vi "sub_ubx-packet-final.vi"(11 "read_buffer":string) -> (1 "ubx arr":T1[](array[typedef]) {"class" format="%x"; "id" format="%x"; "len" format="%x"; "payload" format="%02x"; "chksum" format="%02x"; "next" format="%02x"}, 2 "latlong":cluster{dbl, dbl} {"?" format="%.8f"; "?" format="%.8f"}, 3 "val":bool)   [LabVIEW 2019]
uses:
  Ctrl/ubx-packet.ctl
  Ctrl/cmd_common.ctl
panel:
  out "RTK FIXED":bool
  in  "nav":enum32{"HPPOSLLH", "PVT", "DOP"}(tab)
  out "ubx-packet_hpposllh":T1 {"payload" format="%02x"; "chksum" format="%02x"; "next" format="%02x"}
  out "ubx-packet_pvt":T1 {"payload" format="%02x"; "chksum" format="%02x"; "next" format="%02x"}
  out "ubx-packet_dop":T1 {"payload" format="%02x"; "chksum" format="%02x"; "next" format="%02x"}
  out "str":string
  out "RTK FLOAT":bool
  out "flag":bool[](array[boolean])
  out "GNSSfix Type":u8
  out "ubz arr1":T1[](array[typedef]) {"payload" format="%02x"; "chksum" format="%02x"; "next" format="%02x"}
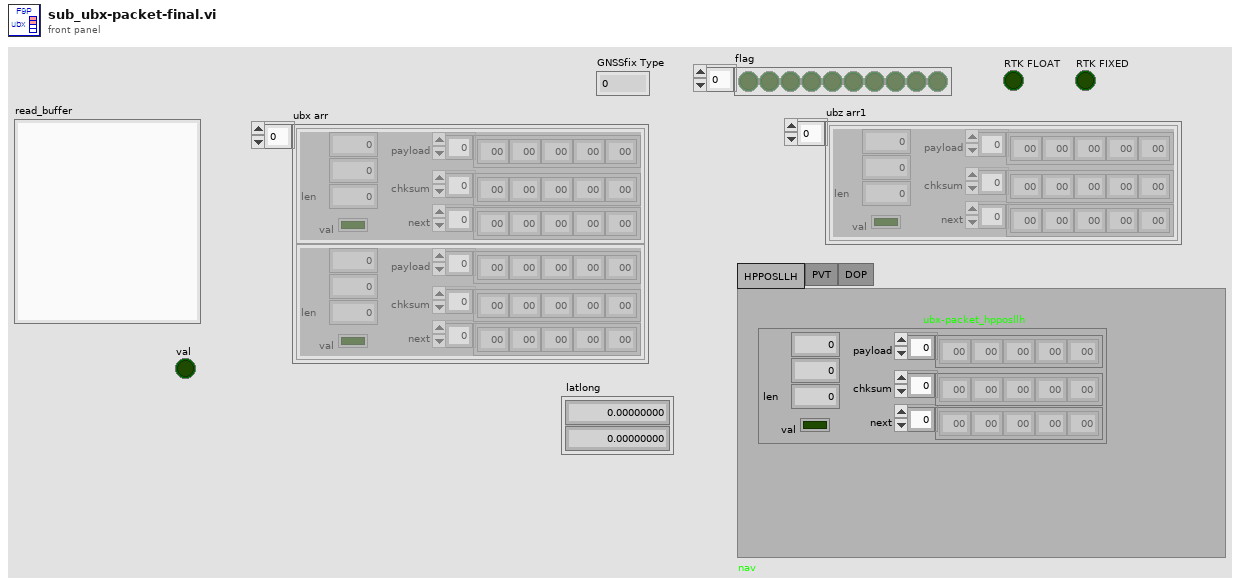
[diagram p1: front panel]
types:
  T1 = typedef "ubx-packet.ctl" = cluster{"class":u8, "id":u8, "len":u8, "payload":u8[], "chksum":u8[], "next ":u8[], "val":bool}
  T2 = typedef "cmd_common.ctl" = enum16{"read", "write"}
  T3 = typedef "ublox-ui_main.ctl" = cluster{"Longitude  ":dbl, "Latitude     ":dbl, "Fix Mode   ":string, "3D Acc.m":dbl, "2D Acc.m":dbl, "PDOP     ":dbl, "HDOP     ":dbl}
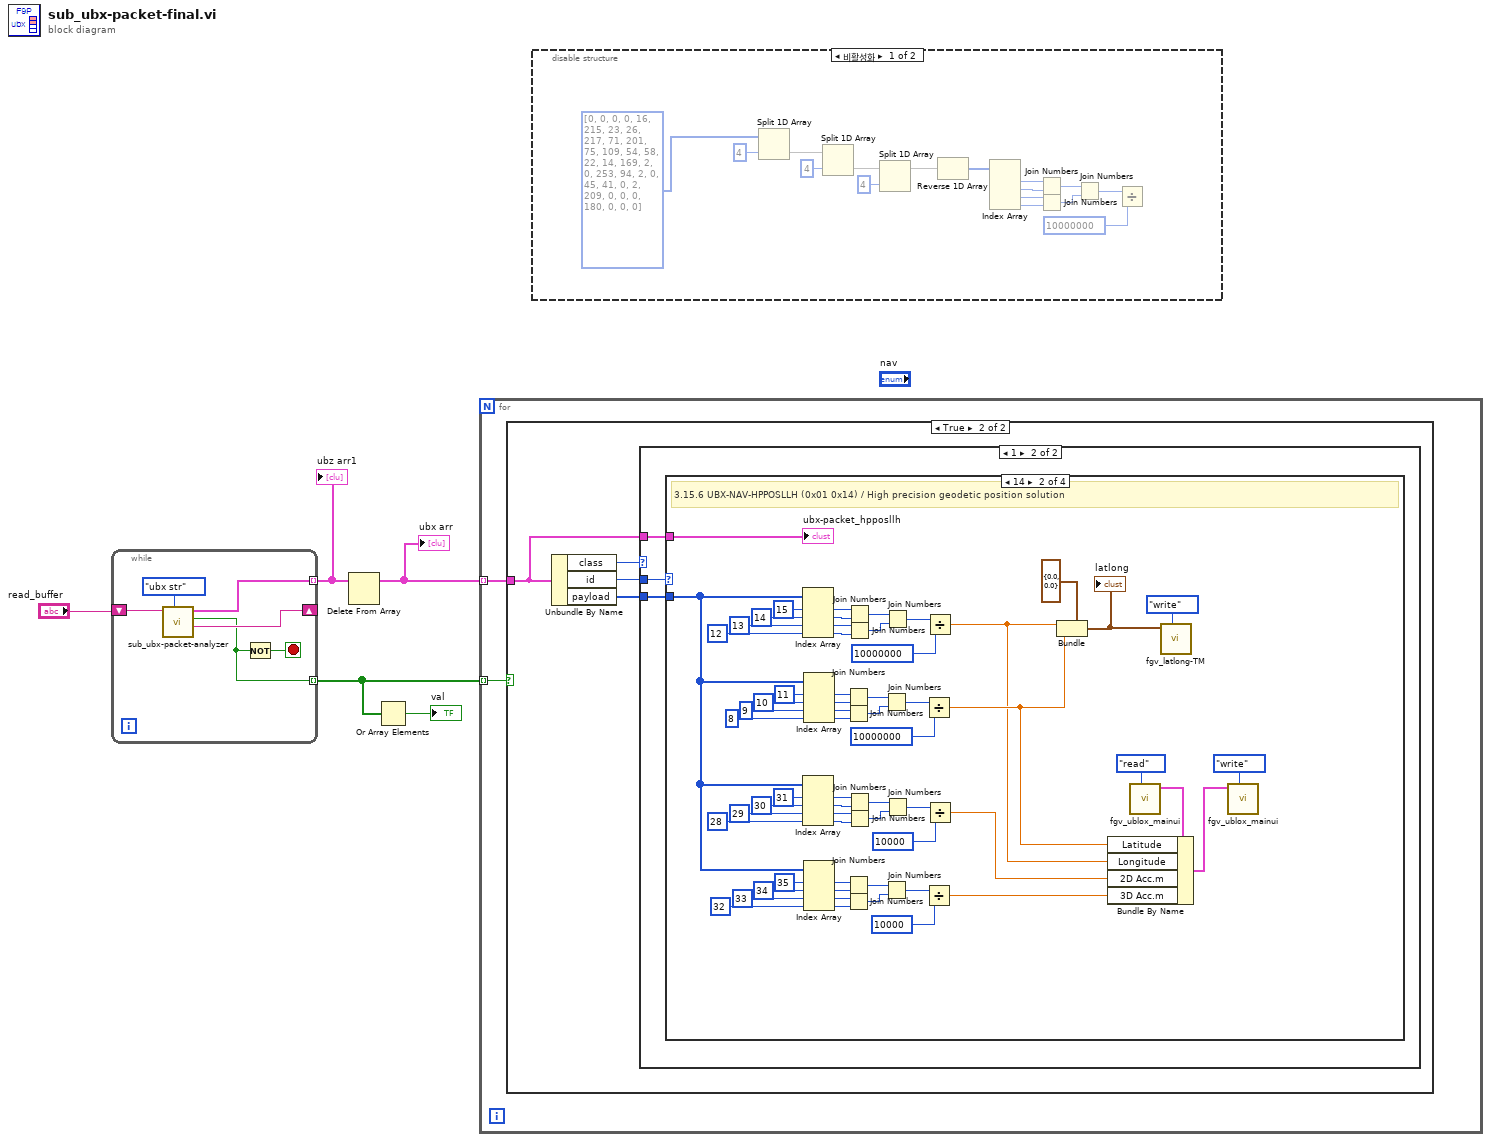
[diagram p0: block diagram]
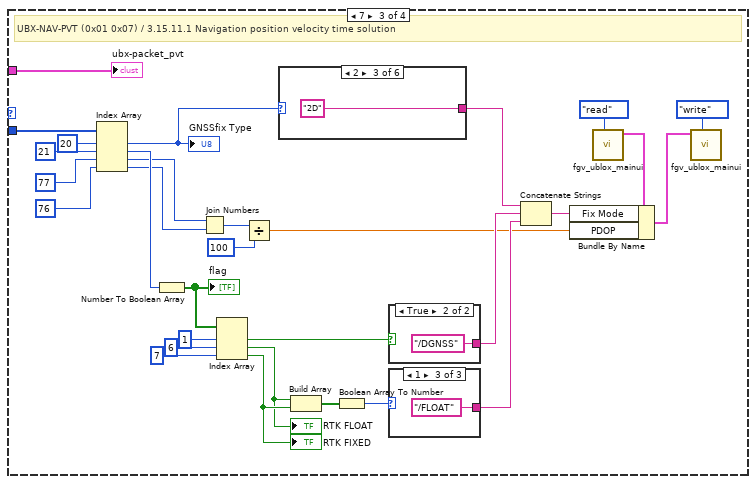
[diagram p5: hidden frame]
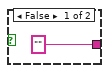
[diagram p6: hidden frame]
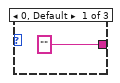
[diagram p7: hidden frame]
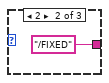
[diagram p8: hidden frame]
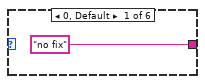
[diagram p9: hidden frame]
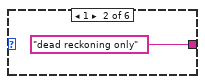
[diagram p10: hidden frame]
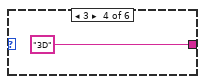
[diagram p11: hidden frame]
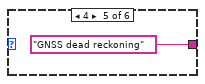
[diagram p12: hidden frame]
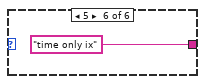
[diagram p13: hidden frame]
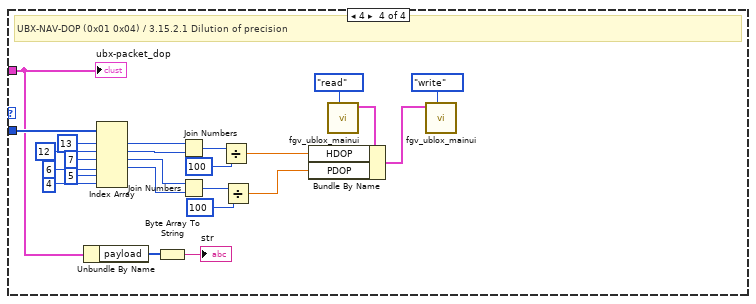
[diagram p14: hidden frame]
diagram:
  n1 = while {
    shift-right: [w8] -> _
    shift-left: "read_buffer" -> [w10]
    tunnel: [w7] -> w5 mode=indexing
    tunnel: [w6] -> w1 mode=indexing
    stop <- w9 stop-if-true
    n2 = call "sub_ubx-packet-analyzer.vi"("cmd"=enum16{"ubx str", "ubx u8arr"}."ubx str", "ubx raw-str"=w10) -> ("next str"=w8:string, "val"=w6:bool, "ubx data"=w7:T1)  [unwired: 7 in]
    n3 = Not(x=w6) -> (.not. x?=w9:bool)
  }
  "ubz arr1" <- w5
  n4 = Delete From Array(array=w5) -> (array with subset deleted=w2:T1[])  [unwired: 2 in, 1 out]
  "ubx arr" <- w2
  n5 = Or Array Elements(Boolean array=w1) -> (logical OR=→"val":bool)
  n6 = for {
    tunnel: w2 -> [w13] mode=indexing
    tunnel: w1 -> [w12] mode=indexing
    n7 = case shown="True" w12 {
      tunnel: w13 -> [_ w14]
      frame False {
      }
      frame True {
        n8 = Unbundle By Name(w14) -> ("class"=w15:u8, "id"=w17:u8, "payload"=w16:u8[])
        n9 = case shown="1" w15 {
          tunnel: w17 -> [_ w20]
          tunnel: w16 -> [_ w19]
          tunnel: w14 -> [_ w18]
          frame 0, Default {
          }
          frame 1 {
            n10 = case shown="14" w20 {
              tunnel: w19 -> [_ w33 w111 w146]
              tunnel: w18 -> [_ w30 w105 w125]
              frame 0, Default {
              }
              frame 20 {
                # "3.15.6 UBX-NAV-HPPOSLLH (0x01 0x14) / High precision geodetic position solution"
                n11 = Index Array(array=w33, index #1=15 ("인덱스"), index #2=14 ("인덱스"), index #3=13 ("인덱스"), index #4=12 ("인덱스")) -> (element #1=w76:u8, element #2=w75:u8, element #3=w77:u8, element #4=w74:u8)
                n12 = Index Array(array=w33, index #1=31 ("인덱스"), index #2=30 ("인덱스"), index #3=29 ("인덱스"), index #4=28 ("인덱스")) -> (element #1=w39:u8, element #2=w40:u8, element #3=w38:u8, element #4=w41:u8)
                n13 = Index Array(array=w33, index #1=11 ("인덱스"), index #2=10 ("인덱스"), index #3=9 ("인덱스"), index #4=8 ("인덱스")) -> (element #1=w62:u8, element #2=w63:u8, element #3=w64:u8, element #4=w65:u8)
                n14 = Index Array(array=w33, index #1=35 ("인덱스"), index #2=34 ("인덱스"), index #3=33 ("인덱스"), index #4=32 ("인덱스")) -> (element #1=w53:u8, element #2=w52:u8, element #3=w51:u8, element #4=w50:u8)
                n15 = Join Numbers(hi=w62, lo=w63) -> ((hi.lo)=w67:u16)
                n16 = Join Numbers(hi=w64, lo=w65) -> ((hi.lo)=w66:u16)
                n17 = Join Numbers(hi=w53, lo=w52) -> ((hi.lo)=w48:u16)
                n18 = Join Numbers(hi=w51, lo=w50) -> ((hi.lo)=w49:u16)
                n19 = Join Numbers(hi=w76, lo=w75) -> ((hi.lo)=w79:u16)
                n20 = Join Numbers(hi=w77, lo=w74) -> ((hi.lo)=w78:u16)
                n21 = Join Numbers(hi=w39, lo=w40) -> ((hi.lo)=w36:u16)
                n22 = Join Numbers(hi=w38, lo=w41) -> ((hi.lo)=w37:u16)
                n23 = Join Numbers(hi=w67, lo=w66) -> ((hi.lo)=w69:u32)
                n24 = Join Numbers(hi=w48, lo=w49) -> ((hi.lo)=w46:u32)
                n25 = Join Numbers(hi=w79, lo=w78) -> ((hi.lo)=w81:u32)
                n26 = Join Numbers(hi=w36, lo=w37) -> ((hi.lo)=w34:u32)
                n27 = Divide(x=w69, y=u32 10000000) -> (x/y=w24:dbl)
                n28 = Divide(x=w46, y=u32 10000) -> (x/y=w22:dbl)
                n29 = Divide(x=w81, y=u32 10000000) -> (x/y=w23:dbl)
                n30 = Divide(x=w34, y=u32 10000) -> (x/y=w25:dbl)
                n31 = Bundle(cluster=cluster{dbl, dbl} {0.0, 0.0} ("출력 클러스터"), w23, w24) -> (w21:cluster{dbl, dbl})
                "latlong" <- w21
                n32 = call "fgv_ublox_mainui.vi"("cmd"=cmd_common."read") -> ("MainUI ublox out"=w27:T3)  [unwired: 10 in]
                n33 = Bundle By Name(cluster=w27, "Latitude"=w24, "Longitude"=w23, "2D Acc.m"=w25, "3D Acc.m"=w22) -> (w26:T3)
                n34 = call "fgv_latlong-TM.vi"("cmd"=enum16{"write", "read"}."write", "latlong"=w21) -> ()  [unwired: 8 in, 2 out]
                n35 = call "fgv_ublox_mainui.vi"("cmd"=cmd_common."write", "MainUI ublox"=w26) -> ()  [unwired: 9 in, 1 out]
                "ubx-packet_hpposllh" <- w30
              }
              frame 7 {
                # "UBX-NAV-PVT (0x01 0x07) / 3.15.11.1 Navigation position velocity time solution"
                n36 = Index Array(array=w111, index #1=20 ("인덱스"), index #2=21 ("인덱스"), index #3=77 ("인덱스"), index #4=76 ("인덱스")) -> (element #1=w103:u8, element #2=w108:u8, element #3=w83:u8, element #4=w82:u8)
                "GNSSfix Type" <- w103
                n37 = Number To Boolean Array(number=w108) -> (Boolean array=w107:bool[])
                "flag" <- w107
                n38 = Join Numbers(hi=w83, lo=w82) -> ((hi.lo)=w86:u16)
                n39 = Index Array(array=w107, index #1=1 ("인덱스"), index #2=6 ("인덱스"), index #3=7 ("인덱스")) -> (element #1=w97:bool, element #2=w101:bool, element #3=w102:bool)
                "RTK FLOAT" <- w101
                "RTK FIXED" <- w102
                n40 = Divide(x=w86, y=u16 100) -> (x/y=w84:dbl)
                n41 = case shown="2" w103 {
                  tunnel: ["no fix" "dead reckoning only" "2D" "3D" "GNSS dead reckoning" "time only ix"] -> w92
                  frame 0, Default {
                  }
                  frame 1 {
                  }
                  frame 2 {
                  }
                  frame 3 {
                  }
                  frame 4 {
                  }
                  frame 5 {
                  }
                }
                n42 = Build Array(w101, w102) -> (w100:bool[])
                n43 = Boolean Array To Number(Boolean array=w100) -> (number=w99:u32)
                n44 = case shown="True" w97 {
                  tunnel: ["" "/DGNSS"] -> w91
                  frame False {
                  }
                  frame True {
                  }
                }
                n45 = case shown="1" w99 {
                  tunnel: ["" "/FIXED" "/FLOAT"] -> w90
                  frame 0, Default {
                  }
                  frame 2 {
                  }
                  frame 1 {
                  }
                }
                n46 = Concatenate Strings(w92, w91, w90) -> (w89:string)
                n47 = call "fgv_ublox_mainui.vi"("cmd"=cmd_common."read") -> ("MainUI ublox out"=w94:T3)  [unwired: 10 in]
                n48 = Bundle By Name(cluster=w94, "Fix Mode"=w89, "PDOP"=w84) -> (w93:T3)
                n49 = call "fgv_ublox_mainui.vi"("cmd"=cmd_common."write", "MainUI ublox"=w93) -> ()  [unwired: 9 in, 1 out]
                "ubx-packet_pvt" <- w105
              }
              frame 4 {
                # "UBX-NAV-DOP (0x01 0x04) / 3.15.2.1 Dilution of precision"
                n50 = Unbundle By Name(w125) -> ("payload"=w124:u8[])
                n51 = Index Array(array=w146, index #1=13 ("인덱스"), index #2=12 ("인덱스"), index #3=7 ("인덱스"), index #4=6 ("인덱스"), index #5=5 ("인덱스"), index #6=4 ("인덱스")) -> (element #1=w135:u8, element #2=w136:u8, element #3=w130:u8, element #4=w129:u8)  [unwired: 2 out]
                n52 = Byte Array To String(unsigned byte array=w124) -> (string=→"str":string)
                n53 = Join Numbers(hi=w135, lo=w136) -> ((hi.lo)=w138:u16)
                n54 = Join Numbers(hi=w130, lo=w129) -> ((hi.lo)=w132:u16)
                n55 = Divide(x=w138, y=u16 100) -> (x/y=w137:dbl)
                n56 = Divide(x=w132, y=u16 100) -> (x/y=w128:dbl)
                n57 = call "fgv_ublox_mainui.vi"("cmd"=cmd_common."read") -> ("MainUI ublox out"=w141:T3)  [unwired: 10 in]
                n58 = Bundle By Name(cluster=w141, "HDOP"=w137, "PDOP"=w128) -> (w140:T3)
                n59 = call "fgv_ublox_mainui.vi"("cmd"=cmd_common."write", "MainUI ublox"=w140) -> ()  [unwired: 9 in, 1 out]
                "ubx-packet_dop" <- w125
              }
            }
          }
        }
      }
    }
  }
  n60 = disable-structure shown="비활성화" {
    frame Disabled {
      n61 = Split 1D Array(array=u8[] [0, 0, 0, 0, 16, 215, 23, 26, 217, 71, 201, 75, 109, 54, 58, 22, 14, 169, 2, 0, 253, 94, 2, 0, 45, 41, 0, 2, 209, 0, 0, 0, 180, 0, 0, 0] ("payload 2"), index=4 ("인덱스")) -> (second subarray=w160:u8[])  [unwired: 1 out]
      n62 = Split 1D Array(array=w160, index=4 ("인덱스")) -> (second subarray=w151:u8[])  [unwired: 1 out]
      n63 = Split 1D Array(array=w151, index=4 ("인덱스")) -> (first subarray=w150:u8[])  [unwired: 1 out]
      n64 = Reverse 1D Array(array=w150) -> (reversed array=w158:u8[])
      n65 = Index Array(array=w158) -> (element #1=w156:u8, element #2=w157:u8, element #3=w155:u8, element #4=w159:u8)  [unwired: 4 in]
      n66 = Join Numbers(hi=w156, lo=w157) -> ((hi.lo)=w153:u16)
      n67 = Join Numbers(hi=w155, lo=w159) -> ((hi.lo)=w154:u16)
      n68 = Join Numbers(hi=w153, lo=w154) -> ((hi.lo)=w148:u32)
      n69 = Divide(x=w148, y=u32 10000000) -> ()  [unwired: 1 out]
    }
    frame Enabled {
    }
  }
